vi "Get Scope Trace.vi"(3 "error in (no error)":errorcluster, 4 "Waveform Source":u16(ring) items=["Ch. 01", "Ch 02", "Ch. 03", "Ch. 04"], 5 "Scope Model":T1=enum."Tek TDS 694C", 6 "Scope Address":refnum<visa-resource-name>) -> (0 "error out":errorcluster, 1 "output waveform":waveform(dbl), 2 "reference out":refnum<visa-resource-name>)   [LabVIEW 2020]
uses:
  Typedefs/Scope Models.ctl
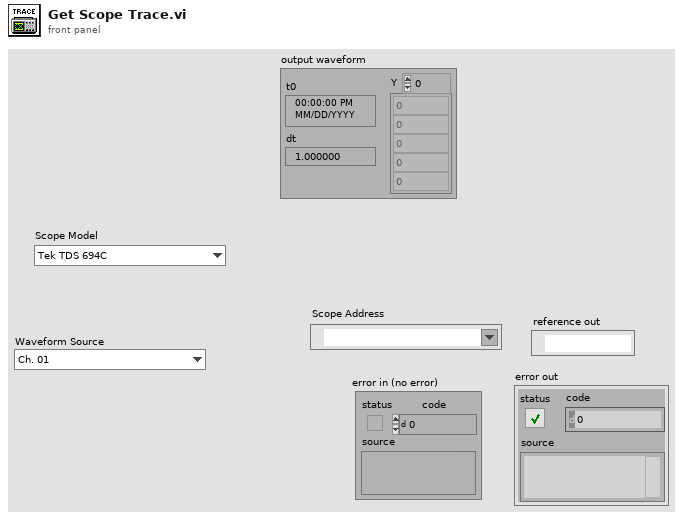
[diagram p1: front panel]
types:
  T1 = typedef "Scope Models.ctl" = enum16{"Tek TDS 684A/B/C", "Tek TDS 694C", "Tek TDS 744/A", "Tek TDS 754A/C/D", "Tek TDS 784A/C/D"}
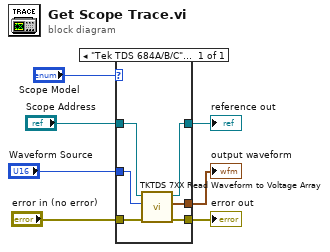
[diagram p0: block diagram]
diagram:
  n1 = case shown="\"Tek TDS 684A/B/C\", Default" "Scope Model" {
    tunnel: "Scope Address" -> [w12]
    tunnel: "error in (no error)" -> [w11]
    tunnel: "Waveform Source" -> [w13]
    tunnel: [w10] -> w3
    tunnel: [w9] -> w2
    tunnel: [w8] -> w1
    frame "Tek TDS 684A/B/C", Default {
      n2 = call <instrlib>:"TKTDS 7XX Read Waveform to Voltage Array.vi"("error in (no error)"=w11, "waveform source (ch1:0)"=w13, "VISA session"=w12) -> ("error out"=w9:errorcluster, "output waveform"=w8:waveform(dbl), "dup VISA session"=w10:refnum<visa-resource-name>)  [unwired: 3 in, 1 out]
    }
  }
  "error out" <- w2
  "reference out" <- w3
  "output waveform" <- w1
